vi "run_td4.vi"() -> ()   [LabVIEW 2025]
uses:
  TD4/TD4.lvclass
  TD4/TD4.lvclass/TD4.ctl
  TD4/ADD A Im.vi
  TD4/ADD B Im.vi
  TD4/MOV A Im.vi
  TD4/MOV B Im.vi
  TD4/MOV A B+Im.vi
  TD4/MOV B A+Im.vi
  TD4/JMP Im.vi
  TD4/JNC Im.vi
  TD4/IN+Im A.vi
  TD4/IN+Im B.vi
  TD4/OUT B+Im.vi
  TD4/OUT Im.vi
  TD4/Increment Program Counter.vi
  TD4/Bool to u8.vi
  TD4/Add with Carry.vi
panel:
  out "Clock":bool
  in  "Stop":bool
  in  "Reset":bool
  in  "Speed":bool
  in  "Input":bool[](array[boolean])
  out "Program Counter":bool[](array[boolean])
  out "Output":bool[](array[boolean])
  out "B":bool[](array[boolean])
  out "A":bool[](array[boolean])
  in  "ROM":bool[][](array[boolean])
  # "TD4 Emulator on LabVIEW"
  # "10Hz"
  # "1Hz"
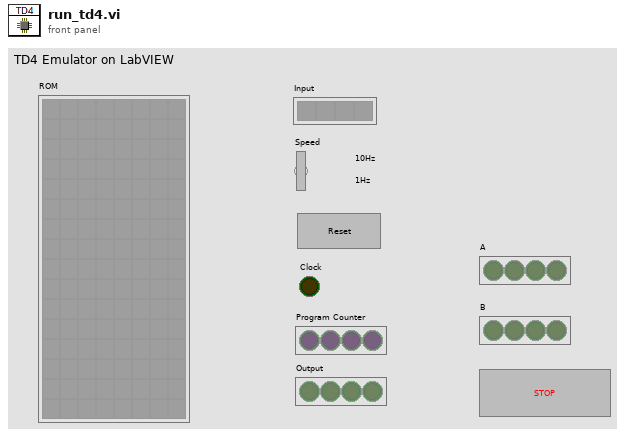
[diagram p1: front panel]
types:
  T1 = typedef "TD4.lvclass/Debug Output.ctl" = cluster{"Program Counter":u8, "A":u8, "B":u8, "Output":u8, "Carry":bool}
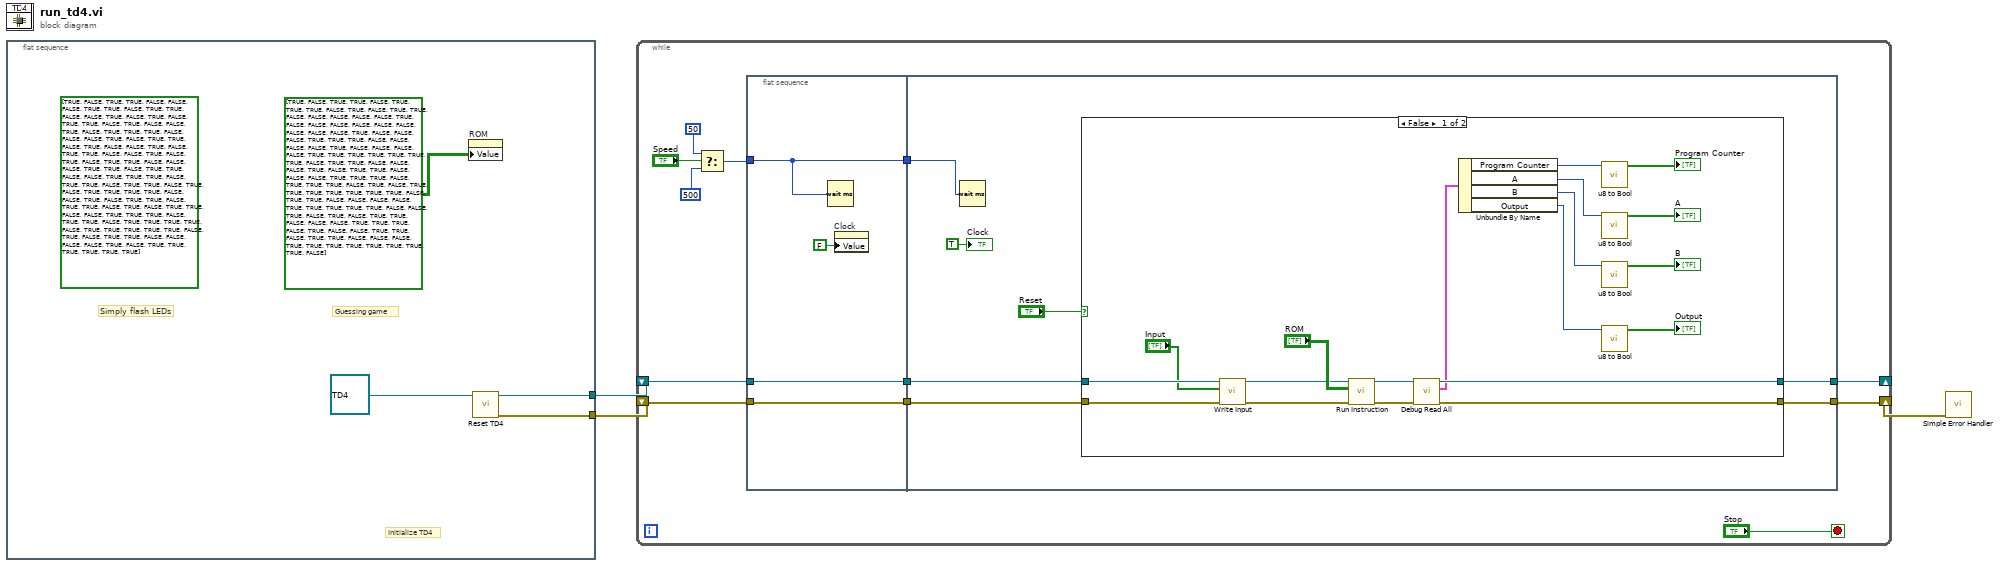
[diagram p0: block diagram]
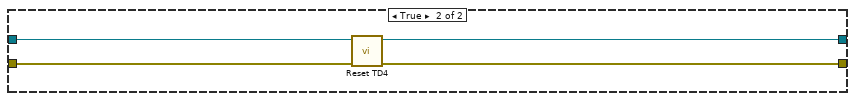
[diagram p2: hidden frame]
diagram:
  n1 = flat-sequence {
    tunnel: [w6] -> w3
    tunnel: [w5] -> w2
    frame #0 {
      (unwired) bool[][] [[TRUE, FALSE, TRUE, TRUE, FALSE, FALSE, FALSE, TRUE], [TRUE, FALSE, TRUE, TRUE, FALSE, FALSE, TRUE, FALSE], [TRUE, FALSE, TRUE, TRUE, FALSE, TRUE, FALSE, FALSE], [TRUE, FALSE, TRUE, TRUE, TRUE, FALSE, FALSE, FALSE], [TRUE, FALSE, TRUE, TRUE, FALSE, TRUE, FALSE, FALSE], [TRUE, FALSE, TRUE, TRUE, FALSE, FALSE, TRUE, FALSE], [TRUE, FALSE, TRUE, TRUE, FALSE, FALSE, FALSE, TRUE], [TRUE, FALSE, TRUE, TRUE, FALSE, FALSE, TRUE, TRUE], [TRUE, FALSE, TRUE, TRUE, FALSE, TRUE, TRUE, FALSE], [TRUE, FALSE, TRUE, TRUE, TRUE, TRUE, FALSE, FALSE], [TRUE, FALSE, TRUE, TRUE, FALSE, TRUE, TRUE, FALSE], [TRUE, FALSE, TRUE, TRUE, FALSE, FALSE, TRUE, TRUE], [TRUE, FALSE, TRUE, TRUE, FALSE, TRUE, TRUE, TRUE], [TRUE, FALSE, TRUE, TRUE, TRUE, TRUE, TRUE, FALSE], [TRUE, FALSE, TRUE, TRUE, FALSE, FALSE, FALSE, FALSE], [TRUE, FALSE, TRUE, TRUE, TRUE, TRUE, TRUE, TRUE]] ("Array")
      # "Guessing game"
      # "Simply flash LEDs"
      # "Initialize TD4"
      n2 = property on="ROM" class="Arr (strict)"("Value"=bool[][] [[TRUE, FALSE, TRUE, TRUE, FALSE, TRUE, TRUE, TRUE], [FALSE, TRUE, FALSE, TRUE, TRUE, FALSE, FALSE, FALSE], [FALSE, FALSE, TRUE, FALSE, FALSE, FALSE, FALSE, FALSE], [FALSE, FALSE, FALSE, FALSE, TRUE, FALSE, FALSE, FALSE], [TRUE, TRUE, TRUE, FALSE, FALSE, FALSE, FALSE, TRUE], [FALSE, FALSE, FALSE, FALSE, TRUE, TRUE, TRUE, TRUE], [TRUE, TRUE, TRUE, FALSE, TRUE, TRUE, FALSE, FALSE], [FALSE, TRUE, FALSE, TRUE, TRUE, FALSE, FALSE, FALSE], [TRUE, TRUE, TRUE, FALSE, TRUE, TRUE, TRUE, FALSE], [TRUE, FALSE, TRUE, TRUE, TRUE, TRUE, TRUE, TRUE], [TRUE, FALSE, TRUE, TRUE, FALSE, FALSE, FALSE, FALSE], [TRUE, TRUE, TRUE, TRUE, TRUE, FALSE, FALSE, TRUE], [FALSE, TRUE, FALSE, TRUE, TRUE, FALSE, FALSE, FALSE], [TRUE, TRUE, TRUE, FALSE, TRUE, FALSE, FALSE, TRUE], [TRUE, FALSE, TRUE, TRUE, FALSE, FALSE, FALSE, TRUE], [TRUE, TRUE, TRUE, TRUE, TRUE, TRUE, TRUE, FALSE]] ("Array")) -> ()  [unwired: 2 in, 2 out]
      n3 = call "Reset TD4.vi"("TD4 in"=refnum<class "TD4.lvclass"> refnum ("TD4.lvclass")) -> ("error out"=w5:errorcluster, "TD4 out"=w6:refnum<class "TD4.lvclass">)  [unwired: 9 in]
    }
  }
  n4 = while {
    shift-right: [w8] -> w1
    shift-left: w2 -> [w10]
    shift-right: [w9] -> _
    shift-left: w3 -> [w12]
    stop <- "Stop" stop-if-true
    n5 = Select(t=u32 50 ("milliseconds to wait"), s="Speed", f=u32 500 ("milliseconds to wait")) -> (s? t:f=w15:u32)
    n6 = flat-sequence {
      tunnel: w15 -> [w23]
      tunnel: [w23] -> w14
      tunnel: [w21] -> w13
      tunnel: w12 -> [w21]
      tunnel: [w20] -> w11
      tunnel: w10 -> [w20]
      tunnel: w14 -> [w30]
      tunnel: w13 -> [w27]
      tunnel: w11 -> [w25]
      tunnel: [w26] -> w9
      tunnel: [w24] -> w8
      frame #0 {
        n7 = Wait (ms)(milliseconds to wait=w23) -> ()  [unwired: 1 out]
        n8 = property on="Clock" class="Bool (strict)"("Value"=FALSE ("Clock")) -> ()  [unwired: 2 in, 2 out]
      }
      frame #1 {
        n9 = Wait (ms)(milliseconds to wait=w30) -> ()  [unwired: 1 out]
        n10 = case shown="False" "Reset" {
          tunnel: w27 -> [w48 w53]
          tunnel: [w41 w52] -> w26
          tunnel: w25 -> [w47 w51]
          tunnel: [w40 w50] -> w24
          frame False {
            n11 = call "Write Input.vi"("error in (no error)"=w47, "Input"="Input", "TD4 in"=w48) -> ("error out"=w45:errorcluster, "TD4 out"=w46:refnum<class "TD4.lvclass">)  [unwired: 7 in]
            n12 = call "Run Instruction.vi"("error in (no error)"=w45, "ROM"="ROM", "TD4 in"=w46) -> ("error out"=w42:errorcluster, "TD4 out"=w43:refnum<class "TD4.lvclass">)  [unwired: 7 in]
            n13 = call "Debug Read All.vi"("error in (no error)"=w42, "TD4 in"=w43) -> ("error out"=w40:errorcluster, "Debug Output"=w39:T1, "TD4 out"=w41:refnum<class "TD4.lvclass">)  [unwired: 7 in]
            n14 = Unbundle By Name(w39) -> ("Program Counter"=w38:u8, "A"=w36:u8, "B"=w35:u8, "Output"=w34:u8)
            n15 = call "u8 to Bool.vi"("Input"=w38) -> ("Output"=→"Program Counter":bool[])  [unwired: 10 in]
            n16 = call "u8 to Bool.vi"("Input"=w36) -> ("Output"=→"A":bool[])  [unwired: 10 in]
            n17 = call "u8 to Bool.vi"("Input"=w35) -> ("Output"=→"B":bool[])  [unwired: 10 in]
            n18 = call "u8 to Bool.vi"("Input"=w34) -> ("Output"=→"Output":bool[])  [unwired: 10 in]
          }
          frame True {
            n19 = call "Reset TD4.vi"("error in (no error)"=w51, "TD4 in"=w53) -> ("error out"=w50:errorcluster, "TD4 out"=w52:refnum<class "TD4.lvclass">)  [unwired: 8 in]
          }
        }
        "Clock" <- TRUE ("Clock")
      }
    }
  }
  n20 = call <vilib>:"Simple Error Handler.vi"("error in (no error)"=w1) -> ()  [unwired: 4 in, 5 out]
